vi "dynamic_datatype_avg_test.vi"() -> ()   [LabVIEW 2021]
panel:
  out "photodiode live avg graph (plots every average, need to update)":cluster{"Y":dbl[], "Y":dbl[]}[](graph)
  out "double array 2":dbl[](array[numeric])
  out "double array":dbl[](array[numeric])
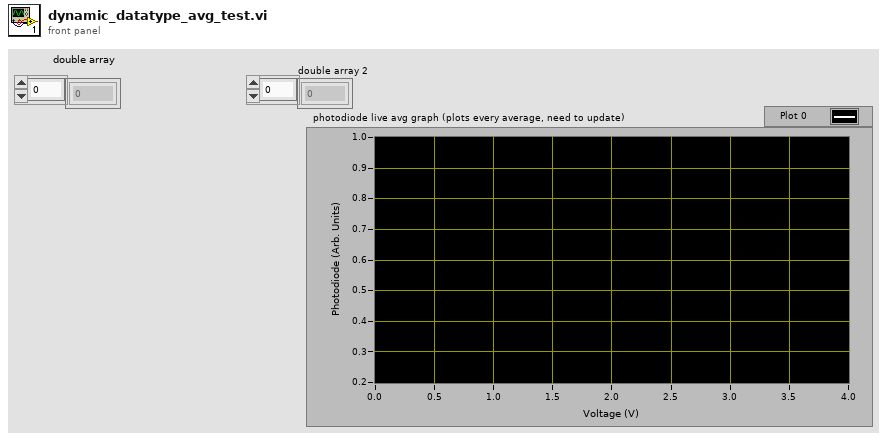
[diagram p1: front panel]
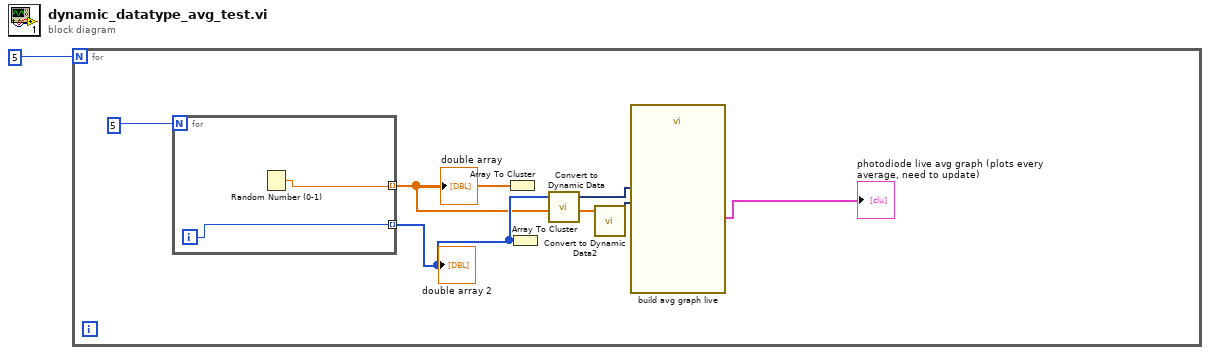
[diagram p0: block diagram]
diagram:
  n1 = for {
    N: 5 -> [_]
    n2 = for {
      N: 5 -> [_]
      tunnel: [w9] -> w5 mode=indexing
      tunnel: [w8] -> w7 mode=indexing
      i -> [w8]
      n3 = Random Number (0-1)() -> (number: 0 to 1=w9:dbl)
    }
    "double array" <- w5
    "double array 2" <- w7
    n4 = Array To Cluster(array=w5) -> ()  [unwired: 1 out]
    n5 = Array To Cluster(array=w7) -> ()  [unwired: 1 out]
    n6 = call "Convert to Dynamic Data"("Array"=w7) -> ("Dynamic Data Type"=w6:dynamicdata)  [unwired: 3 in]
    n7 = call "Convert to Dynamic Data2"("Array"=w5) -> ("Dynamic Data Type"=w4:dynamicdata)  [unwired: 3 in]
    n8 = call "build avg graph live"("Y Input"=w4, "X Input"=w6) -> ("XY Graph"=→"photodiode live avg graph (plots every average, need to update)":cluster{"X":dbl[], "Y":dbl[]}[])  [unwired: 8 in, 1 out]
  }
